vi "Filter Items by Type.vi"(8 "error in (no error)":errorcluster, 11 "CD Build Tools in":refnum<class "Project Build Tools.lvclass">) -> (0 "error out":errorcluster, 1 "Target Names":string[](array[string]), 2 "Build Specifications out":string[](array[string]), 3 "CD Build Tools out":refnum<class "Project Build Tools.lvclass">)   [LabVIEW 2019, in "Project Build Tools.lvclass"]
uses:
  Project Build Tools.lvclass
  Project Build Tools.lvclass/Project Build Tools.ctl
  TypeDefs/Configure Build Types.ctl
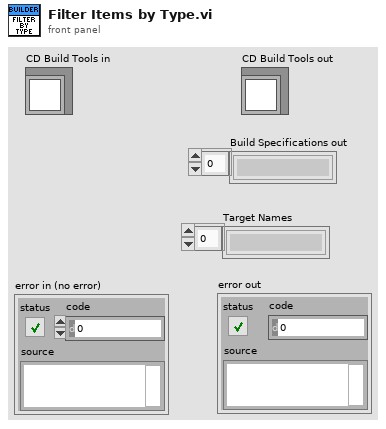
[diagram p1: front panel]
types:
  T1 = typedef "Project Build Tools.lvclass/Configure Build Types.ctl" = enum16{"DLL", "Packed Library", "Installer", "Source Distribution", "EXE"}
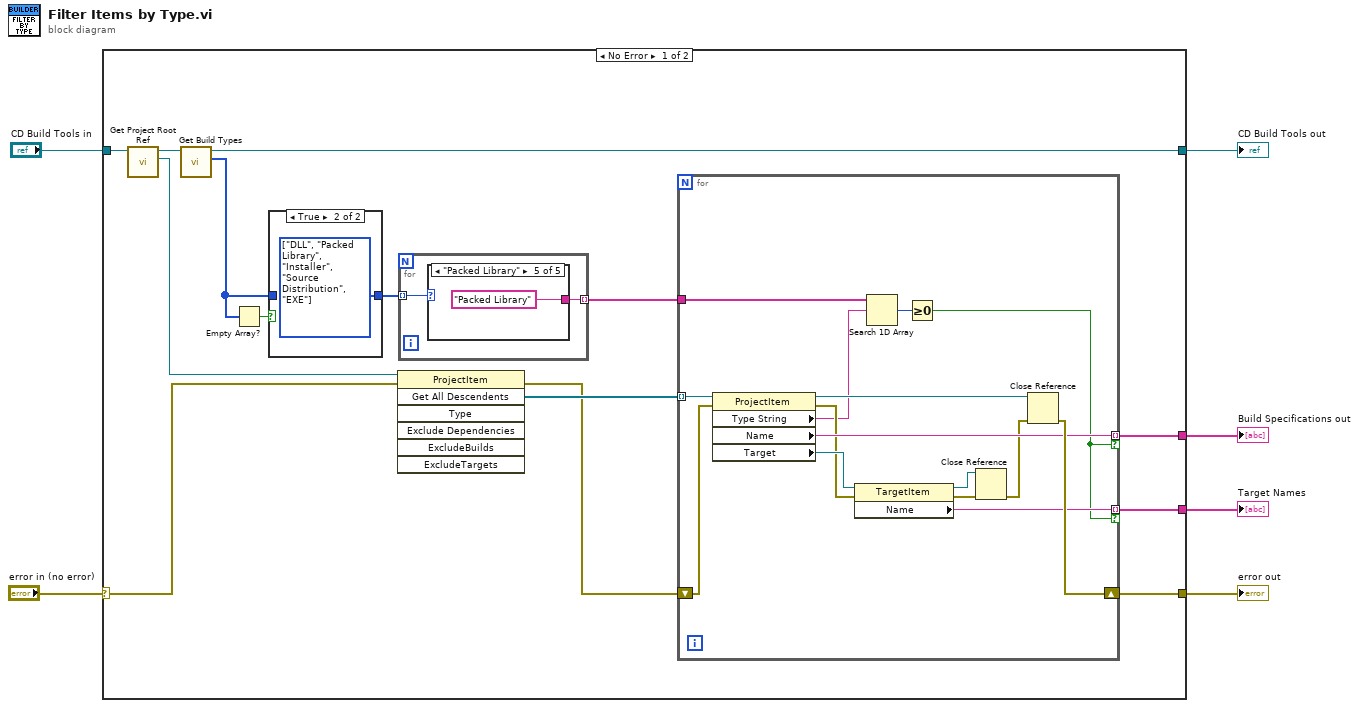
[diagram p0: block diagram]
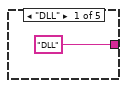
[diagram p3: hidden frame]
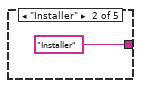
[diagram p4: hidden frame]
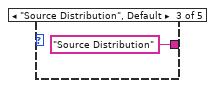
[diagram p5: hidden frame]
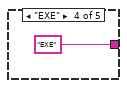
[diagram p6: hidden frame]
diagram:
  n1 = case shown="No Error" "error in (no error)" {
    selector: "error in (no error)" -> [w15 w46]
    tunnel: "CD Build Tools in" -> [w20 w45]
    tunnel: [w19 _] -> w5
    tunnel: [w7 w45] -> w4
    tunnel: [w13 w46] -> w2
    tunnel: [w12 _] -> w1
    frame No Error {
      n2 = call "Get Project Root Ref.vi"("CD Build Tools in"=w20) -> ("Project Root Ref"=w16:refnum<vi>, "CD Build Tools out"=w11:refnum<class "Project Build Tools.lvclass">)  [unwired: 9 in]
      n3 = call "Get Build Types.vi"("CD Build Tools in"=w11) -> ("Build Types"=w9:T1[], "CD Build Tools out"=w7:refnum<class "Project Build Tools.lvclass">)  [unwired: 9 in]
      n4 = Empty Array?(array=w9) -> (empty?=w10:bool)
      n5 = case shown="True" w10 {
        tunnel: w9 -> [w21 _]
        tunnel: [w21 w22] -> w8
        frame False {
        }
        frame True {
          w22 = T1[] [enum."DLL", enum."Packed Library", enum."Installer", enum."Source Distribution", enum."EXE"] items=["DLL", "Packed Library", "Installer", "Source Distribution", "EXE"] ("Build Types")
        }
      }
      n6 = invoke class="ProjectItem" method="Get All Descendents"(reference=w16, error in=w15) -> (error out=w14:errorcluster, "All Descendents"=w17:refnum<vi>[])  [unwired: 5 in, 5 out]
      n7 = for {
        tunnel: [w39] -> w18 mode=indexing
        tunnel: w8 -> [w38] mode=indexing
        n8 = case shown="\"Packed Library\"" w38 {
          tunnel: ["DLL" "Installer" "Source Distribution" "EXE" "Packed Library"] -> w39
          frame "DLL" {
          }
          frame "Installer" {
          }
          frame "Source Distribution", Default {
          }
          frame "EXE" {
          }
          frame "Packed Library" {
          }
        }
      }
      n9 = for {
        tunnel: w17 -> [w37] mode=indexing
        tunnel: w18 -> [w36]
        tunnel: [w31] -> w19 mode=indexing if=w23
        shift-right: [w34] -> w13
        shift-left: w14 -> [w30]
        tunnel: [w28] -> w12 mode=indexing if=w23
        n10 = property class="ProjectItem"(reference=w37, error in=w30) -> (reference out=w33:refnum<vi>, error out=w29:errorcluster, "Type String"=w24:string, "Name"=w31:string, "Target"=w32:refnum<vi>)
        n11 = property class="TargetItem"(reference=w32, error in=w29) -> (reference out=w26:refnum<vi>, error out=w27:errorcluster, "Name"=w28:string)
        n12 = Search 1D Array(1D array=w36, element=w24) -> (index of element=w35:i32)  [unwired: 1 in]
        n13 = Greater Or Equal To 0?(x=w35) -> (x >= 0?=w23:bool)
        n14 = Close Reference(reference=w26, error in (no error)=w27) -> (error out=w25:errorcluster)
        n15 = Close Reference(reference=w33, error in (no error)=w25) -> (error out=w34:errorcluster)
      }
    }
    frame Error {
    }
  }
  "CD Build Tools out" <- w4
  "Build Specifications out" <- w5
  "error out" <- w2
  "Target Names" <- w1
